vi "Intake Holds Ball (OLD).vi"(9 "time":u32, 10 "motor power":dbl, 11 "PhoenixMotorControlDevRef":T1={"DeviceStatus"={"status"=FALSE, "code"=0, "source"=""}, "Type"=enum."PWM", "PWM"={"PWM Channel"=enum."Invalid", "DeadBand"={"Name"="", "maxPositivePwm"=0, "minPositivePwm"=0, "centerPwm"=0, "maxNegativePwm"=0, "minNegativePwm"=0, "angularRange"=0}}, "CAN"={"Device Number"=0, "SetOutput VI Ref"=variant(enum8{"Percent VBus", "Current", "Speed", "Position", "Voltage"} enum."Percent VBus"), "GetOutput VI Ref"=variant(refnum<k1> refnum), "Enable VI Ref"=variant(dbl 12.0), "Disable VI Ref"=variant(enum8{"Percent VBus", "Speed", "Position", "Slave", "Unchanged / Invalid", "Voltage Compensation", "Current", "Motion Profile"} enum."Percent VBus"), "Data"=variant}, "Invert"=FALSE, "DIO PWM"={"PWM \"Enable\" Channel"=enum."Invalid", "DIOChannel"=enum."Invalid", "PWM Rate"=0.0}}) -> (2 "has ball?":bool)   [LabVIEW 2019]
uses:
  <vilib>/Rock Robotics/WPI/MotorControl/WPI_MotorControlDeviceRef.ctl
  <vilib>/Rock Robotics/WPI/MotorControl/WPI_MotorControlType.ctl
  <vilib>/Rock Robotics/SystemInterfaces/DIO/FPGA_DIOPWMChannel.ctl
  <vilib>/Rock Robotics/WPI/PWM/WPI_PWMDeadband.ctl
  <vilib>/Rock Robotics/SystemInterfaces/DIO/FPGA_DIOChannel.ctl
  <vilib>/Rock Robotics/WPI/ThirdParty/Phoenix-LabVIEW/Motor Controller/Get/CTRE_Phoenix_MotorController_GetSupplyAndStatorCurrent_Enhanced.vi
  <vilib>/ptbypt/NI_PtbyPt.lvlib
panel:
  in  "y":dbl
  out "x .and. y?":bool
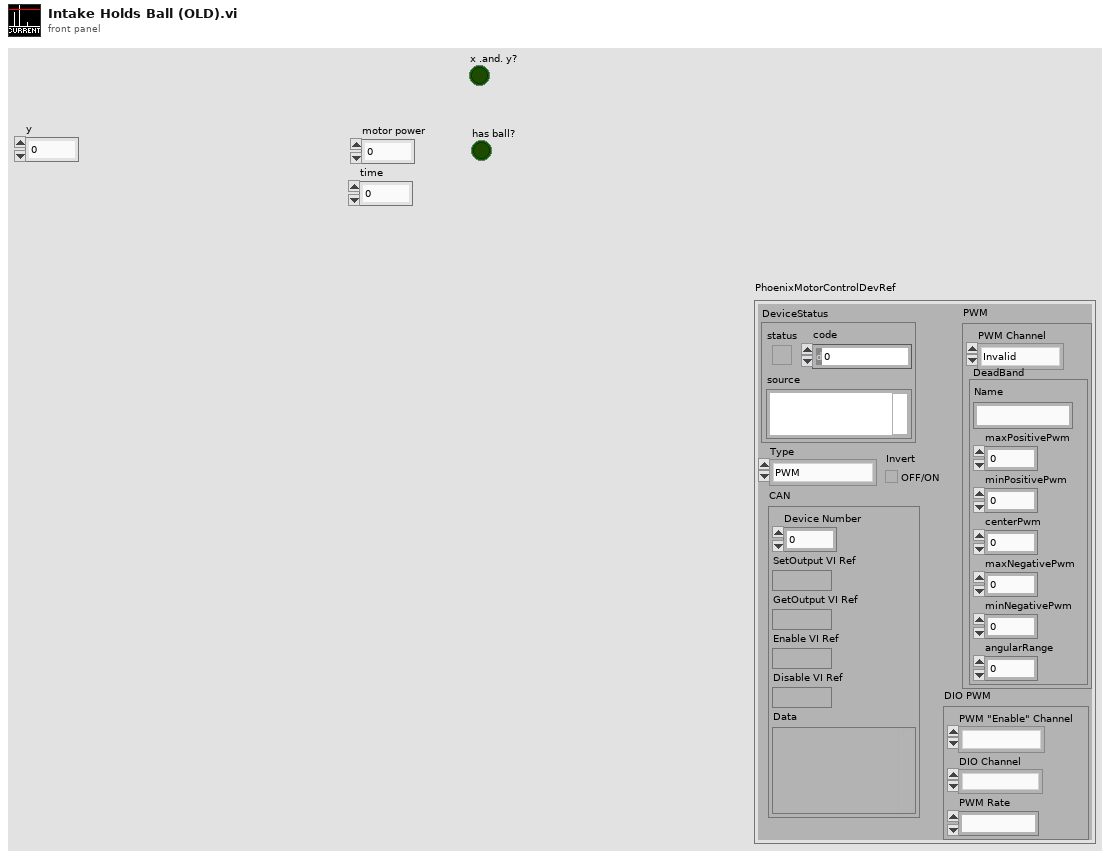
[diagram p1: front panel]
types:
  T1 = typedef "WPI_MotorControlDeviceRef.ctl" = cluster{"DeviceStatus":errorcluster, "Type":T2, "PWM":cluster{"PWM Channel":T3, "DeadBand":T4}, "CAN":cluster{"Device Number":u8, "SetOutput VI Ref":variant, "GetOutput VI Ref":variant, "Enable VI Ref":variant, "Disable VI Ref":variant, "Data":variant}, "Invert":bool, "DIO PWM":cluster{"PWM \"Enable\" Channel":T3, "DIOChannel":T5, "PWM Rate":dbl}}
  T2 = typedef "WPI_MotorControlType.ctl" = enum16{"PWM", "CAN", "DIO PWM"}
  T3 = typedef "FPGA_DIOPWMChannel.ctl" = enum8{"PWM 0", "PWM 1", "PWM 2", "PWM 3", "PWM 4", "PWM 5", "PWM 6", "PWM 7", "PWM 8", "PWM 9", "PWM MXP 0", "PWM MXP 1", "PWM MXP 2", "PWM MXP 3", "PWM MXP 4", "PWM MXP 5", "PWM MXP 6", "PWM MXP 7", "PWM MXP 8", "PWM MXP 9", "Invalid"}
  T4 = typedef "WPI_PWMDeadband.ctl" = cluster{"Name":string, "maxPositivePwm":i32, "minPositivePwm":i32, "centerPwm":i32, "maxNegativePwm":i32, "minNegativePwm":i32, "angularRange":u16}
  T5 = typedef "FPGA_DIOChannel.ctl" = enum8{"DIO 0", "DIO 1", "DIO 2", "DIO 3", "DIO 4", "DIO 5", "DIO 6", "DIO 7", "DIO 8", "DIO 9", "DIO MXP 0", "DIO MXP 1", "DIO MXP 2", "DIO MXP 3", "DIO MXP 4", "DIO MXP 5", "DIO MXP 6", "DIO MXP 7", "DIO MXP 8", "DIO MXP 9", "DIO MXP 10", "DIO MXP 11", "DIO MXP 12", "DIO MXP 13", "DIO MXP 14", "DIO MXP 15", "SPI Port CS1", "SPI Port CS2", "SPI Port CS3", "SPI Port MISO", "SPI Port MOSI", "Invalid"}
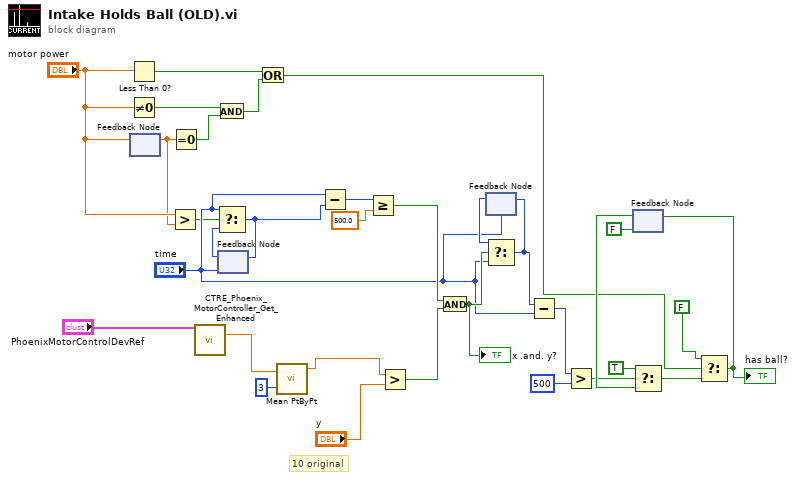
[diagram p0: block diagram]
diagram:
  # "10 original"
  n1 = Less Than 0?(x="motor power") -> (x < 0?=w11:bool)
  n2 = Not Equal To 0?(x="motor power") -> (x != 0?=w8:bool)
  n3 = feedback #1() -> (w5:dbl)  [unwired: 1 in]
  n4 = feedback-in #1("motor power") -> ()
  n5 = Greater?(x="motor power", y=w5) -> (0:w7:bool)
  n6 = Equal To 0?(x=w5) -> (x = 0?=w9:bool)
  n7 = call-poly <vilib>:"CTRE_Phoenix_MotorController_Get_Enhanced.vi"("PhoenixMotorControlDevRef"="PhoenixMotorControlDevRef") -> ("Supply Current"=w31:dbl)  [unwired: 11 in, 3 out]
  n8 = And(x=w8, y=w9) -> (x .and. y?=w10:bool)
  n9 = feedback #2("time") -> (w13:u32)
  n10 = Select(t="time", s=w7, f=w13) -> (s? t:f=w14:u32)
  n11 = feedback-in #2(w14) -> ()
  n12 = Or(x=w11, y=w10) -> (x .or. y?=w3:bool)
  n13 = call <vilib>:"Mean PtByPt.vi"("x"=w31, "sample length"=3) -> ("mean"=w4:dbl)  [unwired: 2 in, 1 out]
  n14 = Subtract(x="time", y=w14) -> (x-y=w16:u32)
  n15 = Greater Or Equal?(x=w16, y=500.0) -> (x >= y?=w15:bool)
  n16 = Greater?(x=w4, y="y") -> (0:w19:bool)
  n17 = And(x=w15, y=w19) -> (x .and. y?=w18:bool)
  "x .and. y?" <- w18
  n18 = feedback #3("time") -> (w23:u32)
  n19 = Select(t=w23, s=w18, f="time") -> (s? t:f=w20:u32)
  n20 = feedback-in #3(w20) -> ()
  n21 = Subtract(x=w20, y="time") -> (x-y=w22:u32)
  n22 = Greater?(x=w22, y=u32 500) -> (0:w21:bool)
  n23 = feedback #4(FALSE ("s")) -> (w28:bool)
  n24 = Select(t=TRUE, s=w21, f=w28) -> (s? t:f=w29:bool)
  n25 = Select(t=FALSE ("s"), s=w3, f=w29) -> (s? t:f=w24:bool)
  "has ball?" <- w24
  n26 = feedback-in #4(w24) -> ()
